vi "tsapp_start_logging_win32.vi"(8 "错误输入（无错误）":errorcluster, 11 "AFileName":string) -> (0 "错误输出":errorcluster, 3 "tsapp_start_logging":i32)   [LabVIEW 2016]
uses:
  TSMaster.dll
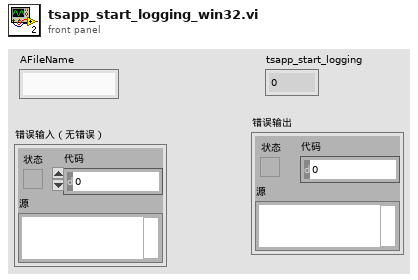
[diagram p1: front panel]
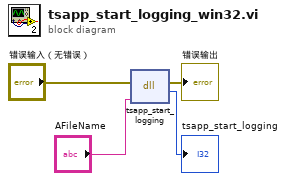
[diagram p0: block diagram]
diagram:
  n1 = dll-call lib="C:/Users/Eric/Desktop/LabVIEW/TSMasterAPI/Win32/CANopen_TS_2015/TSMaster.dll" fn="tsapp_start_logging"(error in="错误输入（无错误）", "AFileName"="AFileName") -> (error out=→"错误输出":errorcluster, "tsapp_start_logging"=→"tsapp_start_logging":i32)  [unwired: 3 in, 1 out]
